vi "Diff Results.vi"(8 "error in (no error)":errorcluster, 10 "RSL Data in":T9 {"Test Config Data"."Test Ranking" items=["Low", "Normal", "High"]}, 11 "Reference RSL Data in":T9 {"Test Config Data"."Test Ranking" items=["Low", "Normal", "High"]}) -> (0 "error out":errorcluster, 3 "RSL Data out":T9 {"Test Config Data"."Test Ranking" items=["Low", "Normal", "High"]})   [LabVIEW 2019]
uses:
  <vilib>/addons/analyzer/_analyzerctrls.llb/VIAnCtl Results.ctl
  <vilib>/addons/analyzer/_analyzerctrls.llb/VIAnCtl ResultsData (index).ctl
  <vilib>/addons/analyzer/_analyzerctrls.llb/VIAnCtl ResultStatus.ctl
  <vilib>/addons/analyzer/_vianresshared.llb/VIAnRes Parsed Results Data (by VI).ctl
  <vilib>/addons/analyzer/_vianresshared.llb/VIAnRes Parsed Results Data (by Test).ctl
  <vilib>/addons/analyzer/_analyzerctrls.llb/VIAnCtl Test Config Data.ctl
  <vilib>/addons/analyzer/_analyzerctrls.llb/VIAnCtl TestRanking.ctl
  <vilib>/addons/analyzer/_analyzerctrls.llb/VIAnCtl Config Control Value.ctl
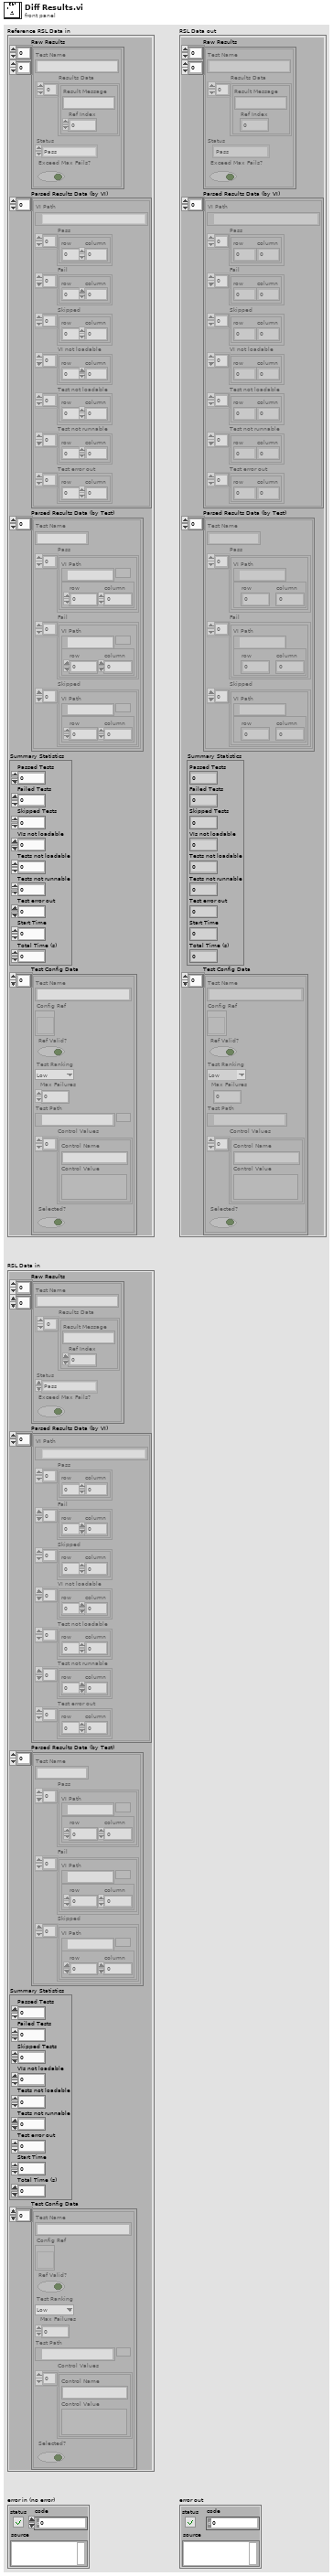
[diagram p1: front panel]
types:
  T1 = typedef "VIAnCtl Results.ctl" = cluster{"Test Name":string, "Results Data":T2[], "Status":T3, "Exceed Max Fails?":bool}
  T2 = typedef "VIAnCtl ResultsData (index).ctl" = cluster{"Result Message":string, "Ref Index":i32}
  T3 = typedef "VIAnCtl ResultStatus.ctl" = enum16{"Pass", "Fail", "Skipped", "VI not loadable", "Test not loadable", "Test not runnable", "Test error out"}
  T4 = typedef "VIAnRes Parsed Results Data (by VI).ctl" = cluster{"VI Path":path, "Pass":cluster{"row":i32, "column":i32}[], "Fail":cluster{"row":i32, "column":i32}[], "Skipped":cluster{"row":i32, "column":i32}[], "VI not loadable":cluster{"row":i32, "column":i32}[], "Test not loadable":cluster{"row":i32, "column":i32}[], "Test not runnable":cluster{"row":i32, "column":i32}[], "Test error out":cluster{"row":i32, "column":i32}[]}
  T5 = typedef "VIAnRes Parsed Results Data (by Test).ctl" = cluster{"Test Name":string, "Pass":cluster{"VI Path":path, "index":cluster{"row":i32, "column":i32}}[], "Fail":cluster{"VI Path":path, "index":cluster{"row":i32, "column":i32}}[], "Skipped":cluster{"VI Path":path, "index":cluster{"row":i32, "column":i32}}[]}
  T6 = typedef "VIAnCtl Test Config Data.ctl" = cluster{"Test Name":string, "Config Ref":refnum<vi>, "Ref Valid?":bool, "Test Ranking":T7, "Max Failures":u32, "Test Path":path, "Control Values":T8[], "Selected?":bool}
  T7 = typedef "VIAnCtl TestRanking.ctl" = u16
  T8 = typedef "VIAnCtl Config Control Value.ctl" = cluster{"Control Name":string, "Control Value":variant}
  T9 = cluster{"Raw Results":T1[][], "Parsed Results Data (by VI)":T4[], "Parsed Results Data (by Test)":T5[], "Summary Statistics":cluster{"Passed Tests":i32, "Failed Tests":i32, "Skipped Tests":i32, "VIs not loadable":i32, "Tests not loadable":i32, "Tests not runnable":i32, "Test error out":i32, "Start Time":u32, "Total Time (s)":dbl}, "Test Config Data":T6[]}
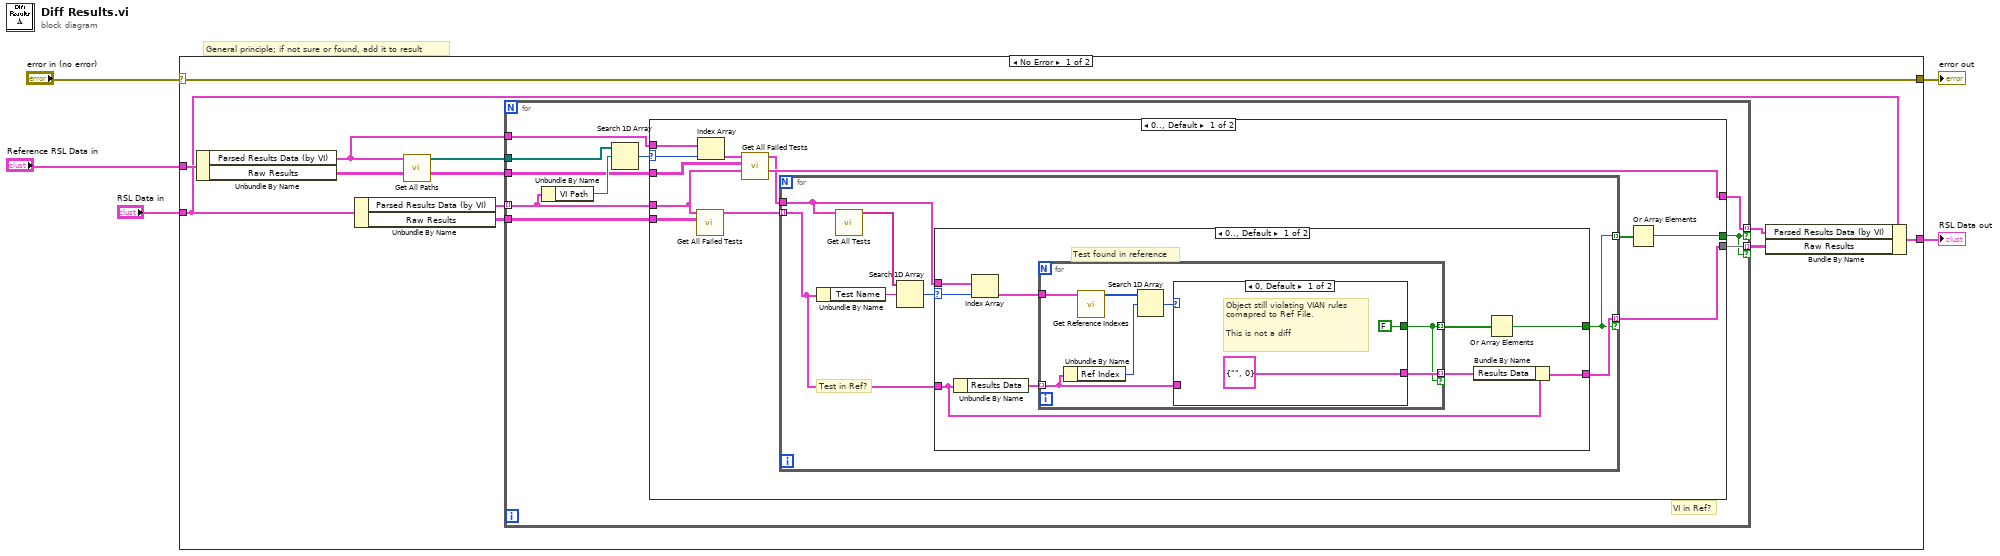
[diagram p0: block diagram]
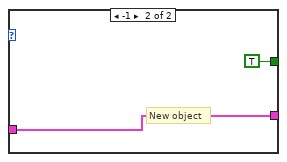
[diagram p2: hidden frame]
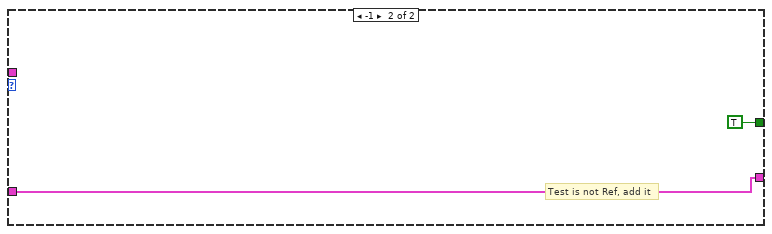
[diagram p3: hidden frame]
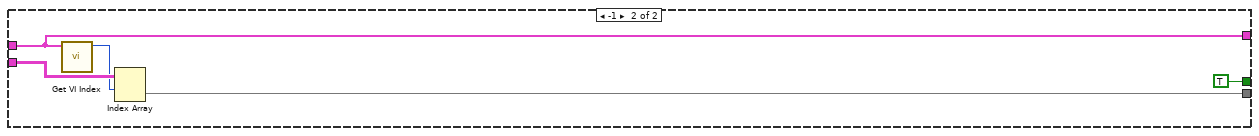
[diagram p4: hidden frame]
diagram:
  # "General principle; if not sure or found, add it to result"
  n1 = case shown="No Error" "error in (no error)" {
    selector: "error in (no error)" -> [w16 w73]
    tunnel: [w16 w73] -> w3
    tunnel: "Reference RSL Data in" -> [w15 w72]
    tunnel: [w11 w72] -> w5
    tunnel: "RSL Data in" -> [w10 _]
    frame No Error {
      n2 = Unbundle By Name(w15) -> ("Parsed Results Data (by VI)"=w8:T4[], "Raw Results"=w6:T1[][])
      n3 = Unbundle By Name(w10) -> ("Parsed Results Data (by VI)"=w13:T4[], "Raw Results"=w12:T1[][])
      n4 = call "Get All Paths.vi"("Parsed Results Data (by VI)"=w8) -> ("Array"=w14:path[])  [unwired: 10 in]
      n5 = for {
        tunnel: w14 -> [w26]
        tunnel: w13 -> [w20] mode=indexing
        tunnel: w12 -> [w23]
        tunnel: [w22] -> w7 mode=indexing if=w19
        tunnel: [w21] -> w9 mode=indexing if=w19
        tunnel: w6 -> [w18]
        tunnel: w8 -> [w17]
        # "VI in Ref?"
        n6 = Unbundle By Name(w20) -> ("VI Path"=w25:path)
        n7 = Search 1D Array(1D array=w26, element=w25) -> (index of element=w24:i32)  [unwired: 1 in]
        n8 = case shown="0.., Default" w24 {
          selector: w24 -> [w36 _]
          tunnel: w23 -> [w35 w69]
          tunnel: [w33 w67] -> w22
          tunnel: [w30 w70] -> w21
          tunnel: w20 -> [w30 w70]
          tunnel: [w31 TRUE] -> w19
          tunnel: w18 -> [w28 _]
          tunnel: w17 -> [w37 _]
          frame 0.., Default {
            n9 = call "Get All Failed Tests.vi"("Raw Results"=w35, "Parsed Results Data (by VI)"=w30) -> ("Failed Tests"=w34:T1[])  [unwired: 9 in]
            n10 = Index Array(array=w37, index=w36) -> (element=w29:T4)
            n11 = call "Get All Failed Tests.vi"("Raw Results"=w28, "Parsed Results Data (by VI)"=w29) -> ("Failed Tests"=w27:T1[])  [unwired: 9 in]
            n12 = for {
              tunnel: w27 -> [w39]
              tunnel: w34 -> [w41] mode=indexing
              tunnel: [w40] -> w33 mode=indexing if=w38
              tunnel: [w38] -> w32 mode=indexing
              # "Test in Ref?"
              n13 = Unbundle By Name(w41) -> ("Test Name"=w43:string)
              n14 = call "Get All Tests.vi"("Array in"=w39) -> ("Test Names"=w44:string[])  [unwired: 10 in]
              n15 = Search 1D Array(1D array=w44, element=w43) -> (index of element=w42:i32)  [unwired: 1 in]
              n16 = case shown="0.., Default" w42 {
                selector: w42 -> [w52 _]
                tunnel: w41 -> [w48 w66]
                tunnel: [w49 w66] -> w40
                tunnel: w39 -> [w53 _]
                tunnel: [w45 TRUE] -> w38
                frame 0.., Default {
                  # "Test found in reference"
                  n17 = Unbundle By Name(w48) -> ("Results Data"=w50:T2[])
                  n18 = Index Array(array=w53, index=w52) -> (element=w51:T1)
                  n19 = for {
                    tunnel: w51 -> [w60]
                    tunnel: w50 -> [w56] mode=indexing
                    tunnel: [w55] -> w47 mode=indexing if=w54
                    tunnel: [w54] -> w46 mode=indexing
                    n20 = Unbundle By Name(w56) -> ("Ref Index"=w58:i32)
                    n21 = call "Get Reference Indexes.vi"("Results"=w60) -> ("Array"=w59:i32[])  [unwired: 10 in]
                    n22 = Search 1D Array(1D array=w59, element=w58) -> (index of element=w57:i32)  [unwired: 1 in]
                    n23 = case shown="0, Default" w57 {
                      tunnel: w56 -> [_ w64]
                      tunnel: [T2 {"Result Message"="", "Ref Index"=0} ("Results Data (index)") w64] -> w55
                      tunnel: [FALSE TRUE] -> w54
                      frame 0, Default {
                        # "Object still violating VIAN rules\ncomapred to Ref File.\n\nThis is not a diff"
                      }
                      frame -1 {
                        # "New object"
                      }
                    }
                  }
                  n24 = Bundle By Name(cluster=w48, "Results Data"=w47) -> (w49:T1)
                  n25 = Or Array Elements(Boolean array=w46) -> (logical OR=w45:bool)
                }
                frame -1 {
                  # "Test is not Ref, add it"
                }
              }
            }
            n26 = Or Array Elements(Boolean array=w32) -> (logical OR=w31:bool)
          }
          frame -1 {
            n27 = call "Get VI Index.vi"("Parsed Results Data (by VI)"=w70) -> ("row"=w68:i32)  [unwired: 10 in]
            n28 = Index Array(array=w69, index (row)=w68) -> (element=w67:T1[])  [unwired: 1 in]
          }
        }
      }
      n29 = Bundle By Name(cluster=w10, "Parsed Results Data (by VI)"=w9, "Raw Results"=w7) -> (w11:T9)
    }
    frame Error {
    }
  }
  "RSL Data out" <- w5
  "error out" <- w3
